vi "Insert Intersection Data In Cluster Array.vi"(8 "ClusterArray":T1(array[cluster]), 9 "Time":dbl, 10 "Y":dbl, 11 "X":dbl) -> (2 "Intersections":T1(array[cluster]))   [LabVIEW 2014]
uses:
  Global FieldWidthY.vi
  Field Class/Global Y Border.vi
  Global FieldLengthX.vi
  Field Class/Global X Border.vi
panel:
  out "upperLimitX":dbl
  out "upperLimitY":dbl
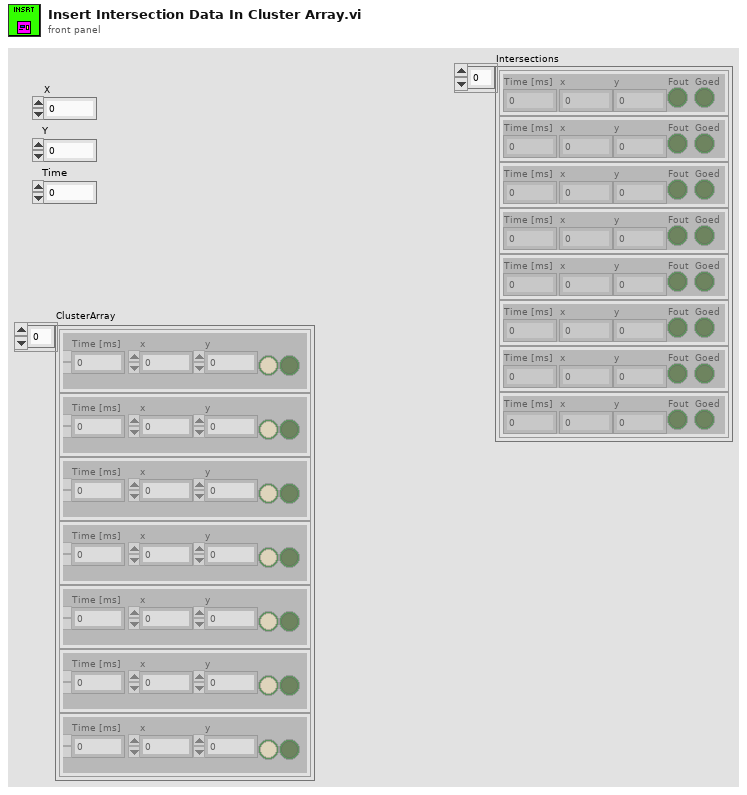
[diagram p1: front panel]
types:
  T1 = cluster{"Time [ms]":dbl, "x":dbl, "y":dbl, "Fout":bool, "Goed":bool}[]
  T2 = cluster{"Time [ms]":dbl, "x":dbl, "y":dbl, "Fout":bool, "Goed":bool}
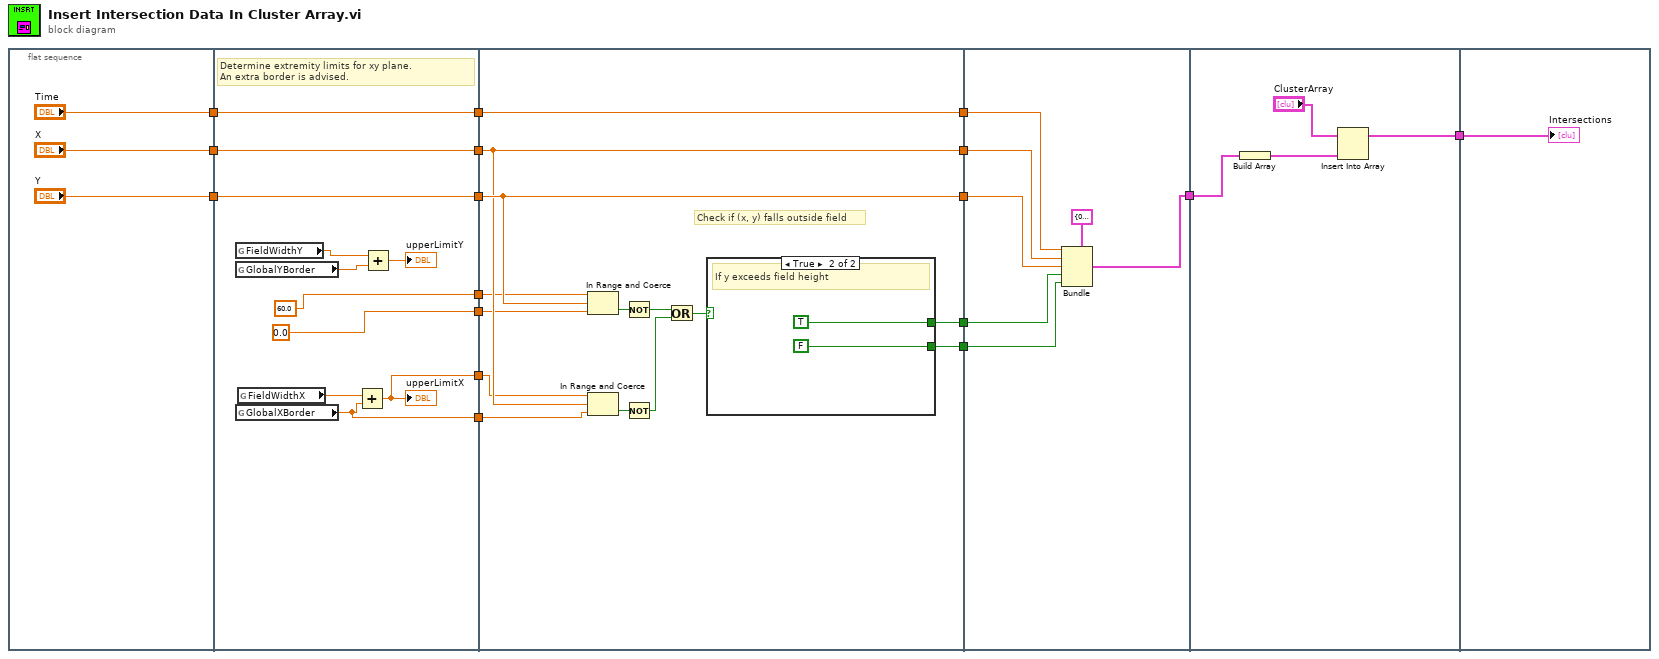
[diagram p0: block diagram]
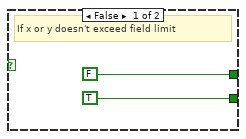
[diagram p2: hidden frame]
diagram:
  n1 = flat-sequence {
    tunnel: ["Time"] -> w10
    tunnel: ["Y"] -> w8
    tunnel: ["X"] -> w6
    tunnel: w10 -> [w31]
    tunnel: [w31] -> w9
    tunnel: w8 -> [w30]
    tunnel: [w30] -> w7
    tunnel: w6 -> [w29]
    tunnel: [w29] -> w5
    tunnel: [60.0] -> w4
    tunnel: [w26] -> w3
    tunnel: [0.0] -> w2
    tunnel: [w23] -> w1
    tunnel: w9 -> [w45]
    tunnel: [w45] -> w16
    tunnel: w7 -> [w42]
    tunnel: [w42] -> w15
    tunnel: [w40] -> w14
    tunnel: w5 -> [w40]
    tunnel: [w44] -> w12
    tunnel: [w43] -> w11
    tunnel: w4 -> [w35]
    tunnel: w3 -> [w34]
    tunnel: w2 -> [w33]
    tunnel: w1 -> [w32]
    tunnel: w16 -> [w56]
    tunnel: w15 -> [w53]
    tunnel: w14 -> [w54]
    tunnel: [w50] -> w13
    tunnel: w12 -> [w52]
    tunnel: w11 -> [w51]
    tunnel: [w59] -> w17
    tunnel: w13 -> [w58]
    tunnel: w17 -> [w61]
    frame #0 {
    }
    frame #1 {
      # "Determine extremity limits for xy plane.\nAn extra border is advised."
      n2 = global read "Global FieldWidthY.vi" "FieldWidthY"() -> (w28:dbl)
      n3 = global read "Global Y Border.vi" "GlobalYBorder"() -> (w24:dbl)
      n4 = global read "Global X Border.vi" "GlobalXBorder"() -> (w23:dbl)
      n5 = global read "Global FieldLengthX.vi" "FieldWidthX"() -> (w25:dbl)
      n6 = Add(x=w25, y=w23) -> (x+y=w26:dbl)
      "upperLimitX" <- w26
      n7 = Add(x=w28, y=w24) -> (x+y=→"upperLimitY":dbl)
    }
    frame #2 {
      # "Check if (x, y) falls outside field"
      n8 = In Range and Coerce(upper limit=w35, x=w42, lower limit=w33) -> (In Range?=w41:bool)  [unwired: 1 out]
      n9 = In Range and Coerce(upper limit=w34, x=w40, lower limit=w32) -> (In Range?=w39:bool)  [unwired: 1 out]
      n10 = Not(x=w41) -> (.not. x?=w37:bool)
      n11 = Not(x=w39) -> (.not. x?=w38:bool)
      n12 = Or(x=w37, y=w38) -> (x .or. y?=w36:bool)
      n13 = case shown="True" w36 {
        tunnel: [FALSE ("Fout") TRUE ("Fout 2")] -> w44
        tunnel: [TRUE ("Goed") FALSE ("Goed")] -> w43
        frame False {
          # "If x or y doesn't exceed field limit"
        }
        frame True {
          # "If y exceeds field height"
        }
      }
    }
    frame #3 {
      n14 = Bundle(cluster=T2 {"Time [ms]"=0.0, "x"=0.0, "y"=0.0, "Fout"=FALSE, "Goed"=FALSE} ("Cluster"), "Time [ms]"=w56, "x"=w54, "y"=w53, "Fout"=w52, "Goed"=w51) -> (w50:T2)
    }
    frame #4 {
      n15 = Build Array "Build Array"(w58) -> (w57:T1)
      n16 = Insert Into Array "Insert Into Array"(array="ClusterArray", new element=w57) -> (w59:T1)  [unwired: 1 in]
    }
    frame #5 {
      "Intersections" <- w61
    }
  }
